vi "IFD RGB Image out.vi"(8 "error in (no error)":errorcluster, 10 "refnum in":refnum<file>, 11 "IFD in":refnum<class "IFD.lvclass">) -> (0 "error out":errorcluster, 2 "refnum out":refnum<file>)   [LabVIEW 2016, in "IFD.lvclass"]
uses:
  IFD.lvclass
  IFD.lvclass/IFD.ctl
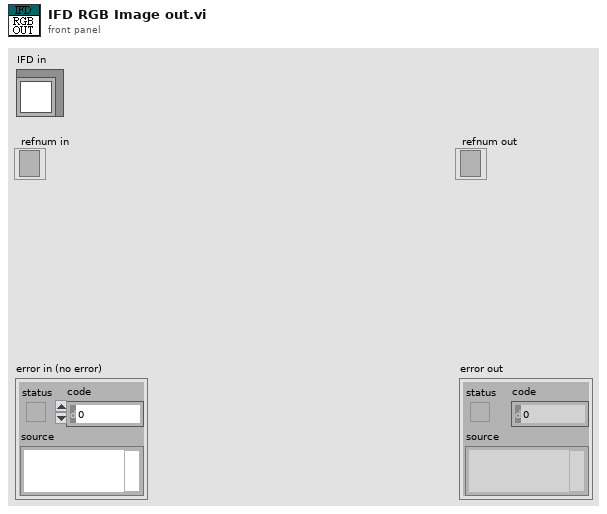
[diagram p1: front panel]
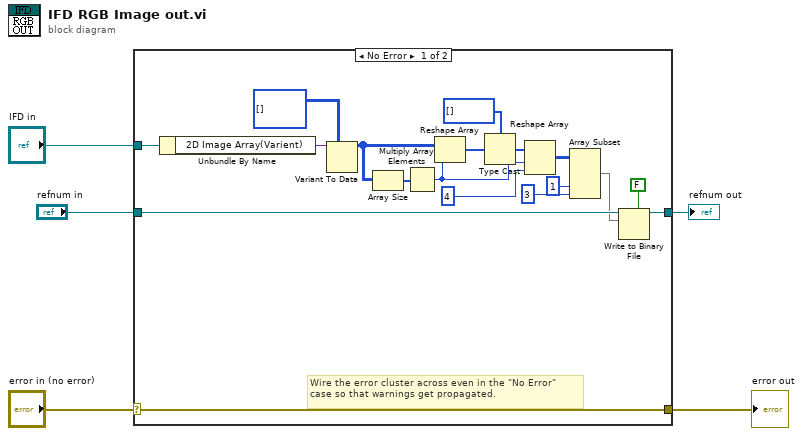
[diagram p0: block diagram]
diagram:
  n1 = case shown="No Error" "error in (no error)" {
    selector: "error in (no error)" -> [w23 w25]
    tunnel: [w23 w25] -> w4
    tunnel: "IFD in" -> [w22 _]
    tunnel: [w19 w24] -> w2
    tunnel: "refnum in" -> [w18 w24]
    frame No Error {
      # "Wire the error cluster across even in the \"No Error\"\ncase so that warnings get propagated."
      n2 = Unbundle By Name(w22) -> ("2D Image Array(Varient)"=w21:variant)
      n3 = Variant To Data(type=u32[][] [], Variant=w21) -> (data=w14:u32[][])  [unwired: 1 in, 1 out]
      n4 = Array Size(array=w14) -> (size(s)=w13:i32[])
      n5 = Multiply Array Elements(1:w13) -> (0:w8:i32)
      n6 = Reshape Array(w14, w8) -> (w15:u32[])
      n7 = Type Cast(type=u8[] [], x=w15) -> (*(type *) &x=w9:u8[])
      n8 = Reshape Array(w9, w8, 4 ("dimension size")) -> (w12:u8[][])
      n9 = Array Subset(array=w12, index (col)=1 ("index"), length (col)=3 ("length")) -> (w6:u8[][])  [unwired: 2 in]
      n10 = Write to Binary File(file (use dialog)=w18, data=w6, 5:FALSE ("prepend array or string size? (T)")) -> (refnum out=w19:refnum<file>)  [unwired: 3 in, 2 out]
    }
    frame Error {
    }
  }
  "error out" <- w4
  "refnum out" <- w2
